vi "Get Range Values[].vi"(0 "Start":dbl, 5 "Stop":dbl, 7 "Step Size":dbl) -> (4 "Values[]":dbl[](array[numeric]))   [LabVIEW 2020]
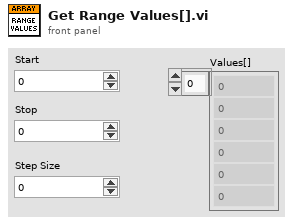
[diagram p1: front panel]
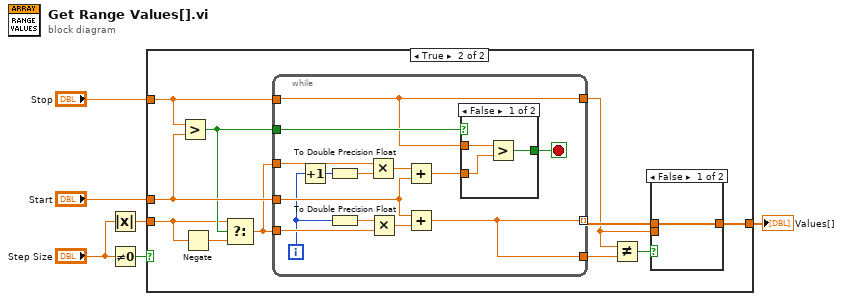
[diagram p0: block diagram]
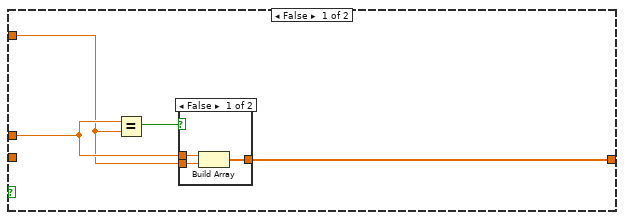
[diagram p2: hidden frame]
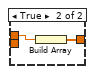
[diagram p3: hidden frame]
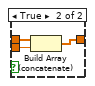
[diagram p4: hidden frame]
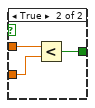
[diagram p5: hidden frame]
diagram:
  n1 = Absolute Value(x="Step Size") -> (abs(x)=w5:dbl)
  n2 = Not Equal To 0?(x="Step Size") -> (x != 0?=w6:bool)
  n3 = case shown="True" w6 {
    tunnel: "Start" -> [w9 w26]
    tunnel: "Stop" -> [w8 w25]
    tunnel: [w10 w18] -> w1
    tunnel: w5 -> [_ w16]
    frame False {
      n4 = Equal?(x=w9, y=w8) -> (x = y?=w7:bool)
      n5 = case shown="False" w7 {
        tunnel: [w13 w15] -> w10
        tunnel: w9 -> [w12 w14]
        tunnel: w8 -> [w11 _]
        frame False {
          n6 = Build Array(w12, w11) -> (w13:dbl[])
        }
        frame True {
          n7 = Build Array(w14) -> (w15:dbl[])
        }
      }
    }
    frame True {
      n8 = Greater?(x=w25, y=w26) -> (0:w19:bool)
      n9 = Negate(x=w16) -> (-x=w24:dbl)
      n10 = Select(t=w16, s=w19, f=w24) -> (s? t:f=w23:dbl)
      n11 = while {
        tunnel: w26 -> [w40]
        tunnel: w25 -> [w35]
        tunnel: w23 -> [w44]
        tunnel: [w36] -> w21 mode=indexing
        tunnel: w19 -> [w43]
        tunnel: w23 -> [w37]
        tunnel: [w36] -> w22
        tunnel: [w35] -> w20
        i -> [w31]
        stop <- w41 stop-if-true
        n12 = Increment(x=w31) -> (x+1=w34:i32)
        n13 = To Double Precision Float(number=w34) -> (double precision float=w33:dbl)
        n14 = To Double Precision Float(number=w31) -> (double precision float=w32:dbl)
        n15 = Multiply(x=w44, y=w33) -> (x*y=w39:dbl)
        n16 = Multiply(x=w32, y=w37) -> (x*y=w38:dbl)
        n17 = Add(x=w39, y=w40) -> (x+y=w42:dbl)
        n18 = Add(x=w40, y=w38) -> (x+y=w36:dbl)
        n19 = case shown="False" w43 {
          tunnel: w42 -> [w45 w49]
          tunnel: w35 -> [w47 w50]
          tunnel: [w46 w48] -> w41
          frame False {
            n20 = Greater?(x=w47, y=w45) -> (0:w46:bool)
          }
          frame True {
            n21 = Less?(x=w50, y=w49) -> (x < y?=w48:bool)
          }
        }
      }
      n22 = Not Equal?(x=w20, y=w22) -> (x != y?=w17:bool)
      n23 = case shown="False" w17 {
        tunnel: w20 -> [_ w30]
        tunnel: w21 -> [w27 w29]
        tunnel: [w27 w28] -> w18
        frame False {
        }
        frame True {
          n24 = Build Array (concatenate)(w29, w30) -> (w28:dbl[])
        }
      }
    }
  }
  "Values[]" <- w1
